vi "HV Create OnStates.vi"(11 "Voltages":string[](array[string])) -> (3 "Onstates":string[](array[string]))   [LabVIEW 2018, in "HV QMH.lvlib"]
uses:
  HV QMH.lvlib
panel:
  # "Decides which channels should be turned on/off based on which elements in array are non-zero"
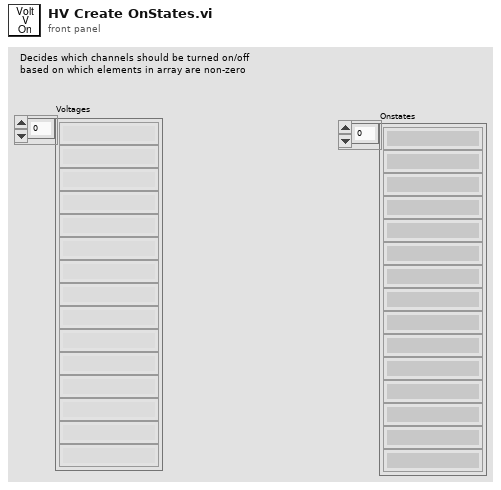
[diagram p1: front panel]
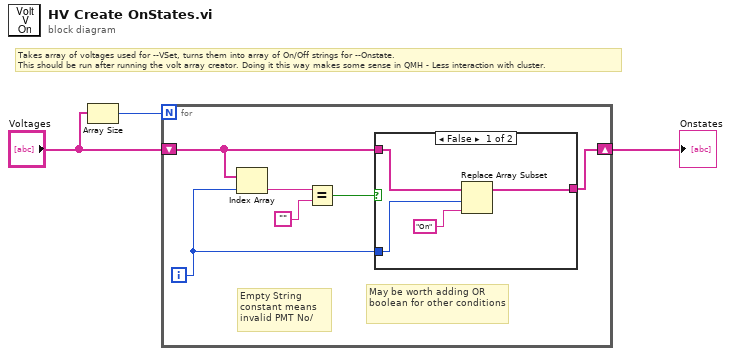
[diagram p0: block diagram]
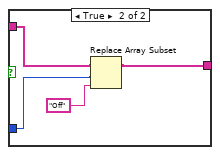
[diagram p2: hidden frame]
diagram:
  # "Takes array of voltages used for --VSet, turns them into array of On/Off strings for --Onstate.\nThis should be run after running the volt array creator. Doing it this way makes some sense in QMH - Less interaction with cluster."
  n1 = Array Size(array="Voltages") -> (size(s)=w2:i32)
  n2 = for {
    N: w2 -> [_]
    shift-right: [w4] -> w1
    shift-left: "Voltages" -> [w5]
    i -> [w6]
    # "May be worth adding OR boolean for other conditions"
    # "Empty String constant means invalid PMT No/"
    n3 = Index Array(array=w5, index=w6) -> (element=w8:string)
    n4 = Equal?(x=w8, y="") -> (x = y?=w7:bool)
    n5 = case shown="False" w7 {
      tunnel: w6 -> [w10 w15]
      tunnel: w5 -> [w12 w17]
      tunnel: [w13 w16] -> w4
      frame False {
        n6 = Replace Array Subset(array=w12, new element="On", index=w10) -> (w13:string[])
      }
      frame True {
        n7 = Replace Array Subset(array=w17, new element="Off", index=w15) -> (w16:string[])
      }
    }
  }
  "Onstates" <- w1
